vi "AG34980A_Configure_Frequency_and_Period.vi"(0 "VISA resource name":refnum<visa-resource-name>, 5 "Mode":enum16{"Frequency", "Period"}(ring)=enum."Period", 7 "Voltage Range (5:Auto)":T3(ring)=enum."Auto", 9 "Low Frequency (1:20 Hz)":T2(ring)=enum."20 Hz", 11 "error in (no error)":errorcluster, 12 "Aperture (1:100 ms)":T1(ring)=enum."100 ms") -> (4 "VISA resource name out":refnum<visa-resource-name>, 15 "error out":errorcluster)   [LabVIEW 2022 SP3, in "DMM_Keysight_34980A.lvlib" / "DMM_Keysight_34980A.lvclass"]
doc: "This VI allows you to configure various settings for performing frequency and period measurements. The VI can be usedt to set the voltage range, the low frequency, and the aperture time. The Channel List parameter can be used to configure multiple channels at once."
uses:
  DMM_Keysight_34980A.lvclass
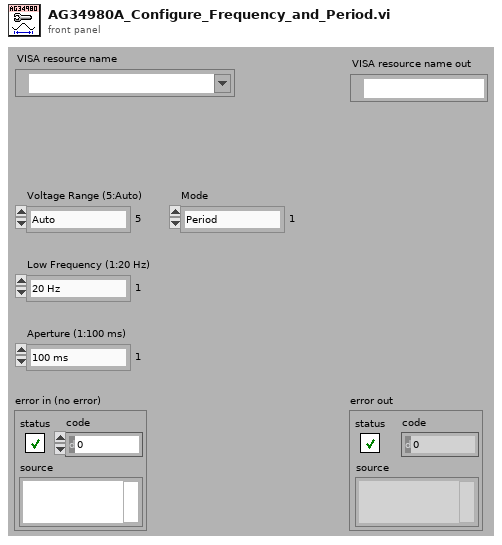
[diagram p1: front panel]
types:
  T1 = enum16{"10 ms", "100 ms", "1 sec", "Minimum", "Maximum"}
  T2 = enum16{"3 Hz", "20 Hz", "200 Hz", "Minimum", "Maximum"}
  T3 = enum16{"100 mV", "1 V", "10 V", "100 V", "300 V", "Auto", "Minimum", "Maximum"}
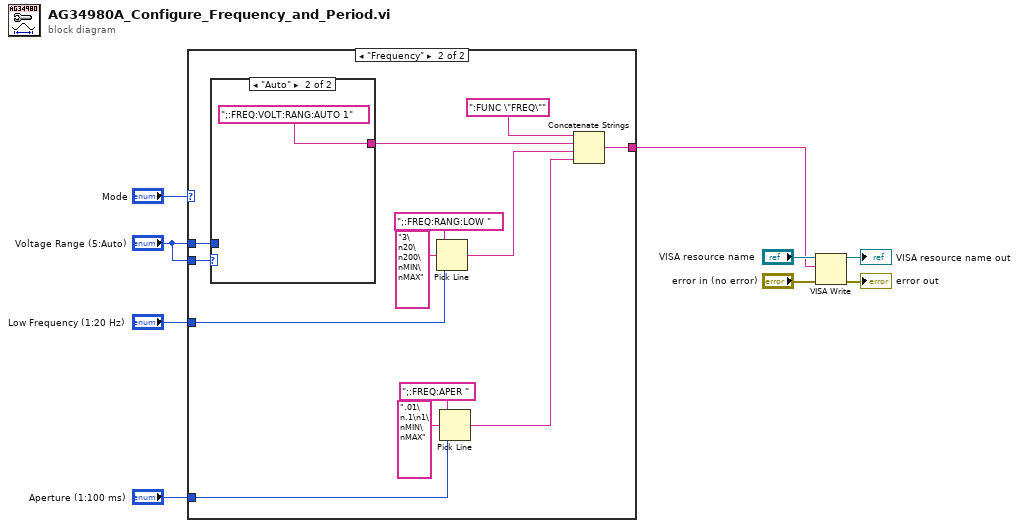
[diagram p0: block diagram]
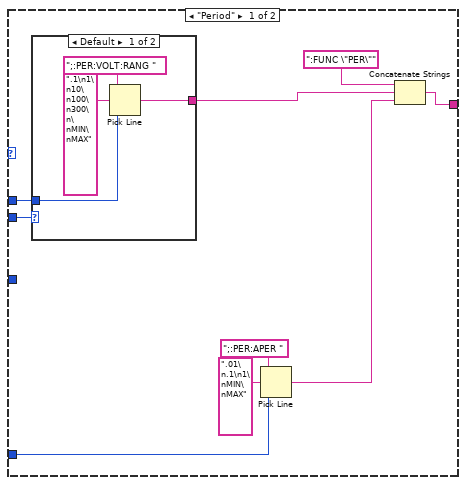
[diagram p2: hidden frame]
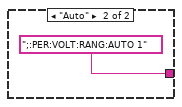
[diagram p3: hidden frame]
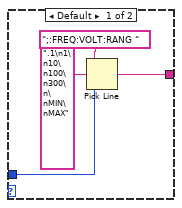
[diagram p4: hidden frame]
diagram:
  n1 = case shown="\"Frequency\"" "Mode" {
    tunnel: "Voltage Range (5:Auto)" -> [w18 w36]
    tunnel: "Low Frequency (1:20 Hz)" -> [_ w34]
    tunnel: "Aperture (1:100 ms)" -> [w13 w27]
    tunnel: [w12 w26] -> w3
    tunnel: "Voltage Range (5:Auto)" -> [w11 w25]
    frame "Period" {
      n2 = case shown="Default" w18 {
        tunnel: [w20 ";:PER:VOLT:RANG:AUTO 1"] -> w17
        tunnel: w11 -> [w19 _]
        frame Default {
          n3 = Pick Line(string ("")=";:PER:VOLT:RANG ", multi-line string=".1\n1\n10\n100\n300\n\nMIN\nMAX", line index=w19) -> (output string=w20:string)
        }
        frame "Auto" {
        }
      }
      n4 = Pick Line(string ("")=";:PER:APER ", multi-line string=".01\n.1\n1\nMIN\nMAX", line index=w13) -> (output string=w14:string)
      n5 = Concatenate Strings(":FUNC \"PER\"", w17, w14) -> (w12:string)
    }
    frame "Frequency" {
      n6 = case shown="\"Auto\"" w36 {
        tunnel: [w38 ";:FREQ:VOLT:RANG:AUTO 1"] -> w33
        tunnel: w25 -> [w37 _]
        frame Default {
          n7 = Pick Line(string ("")=";:FREQ:VOLT:RANG ", multi-line string=".1\n1\n10\n100\n300\n\nMIN\nMAX", line index=w37) -> (output string=w38:string)
        }
        frame "Auto" {
        }
      }
      n8 = Pick Line(string ("")=";:FREQ:RANG:LOW ", multi-line string="3\n20\n200\nMIN\nMAX", line index=w34) -> (output string=w29:string)
      n9 = Pick Line(string ("")=";:FREQ:APER ", multi-line string=".01\n.1\n1\nMIN\nMAX", line index=w27) -> (output string=w28:string)
      n10 = Concatenate Strings(":FUNC \"FREQ\"", w33, w29, w28) -> (w26:string)
    }
  }
  n11 = VISA Write(VISA resource name="VISA resource name", write buffer=w3, error in (no error)="error in (no error)") -> (VISA resource name out=→"VISA resource name out":refnum<visa-resource-name>, error out=→"error out":errorcluster)  [unwired: 1 out]
